vi "AutoSwitchCaptSimu.vi"() -> ()   [LabVIEW 2012]
panel:
  in  "AutoSwitchCaptSimu":bool
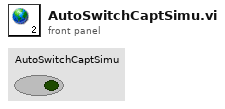
[diagram p1: front panel]
diagram:
